vi "Run 2 Averaged History.vi"(11 "2D Run Data":dbl[][](array[numeric])=[[1.0, 11.0], [2.0, 12.0], [3.0, 13.0], [4.0, 14.0], [5.0, 15.0], [6.0, 16.0], [7.0, 17.0], [8.0, 18.0], [9.0, 19.0], [10.0, 20.0], [2.0, 12.0], [3.0, 13.0], [4.0, 14.0], [5.0, 15.0], [6.0, 16.0], [7.0, 17.0], [8.0, 18.0], [9.0, 19.0], [10.0, 20.0], [11.0, 21.0]]) -> (3 "Data 2D IN out":dbl[](array[numeric]))   [LabVIEW 2011]
panel:
  out "Averaged Integration Spectra":dbl[][](array[numeric])=[[1.5, 11.5], [2.5, 12.5], [3.5, 13.5], [4.5, 14.5], [5.5, 15.5], [6.5, 16.5], [7.5, 17.5], [8.5, 18.5], [9.5, 19.5], [10.5, 20.5]]
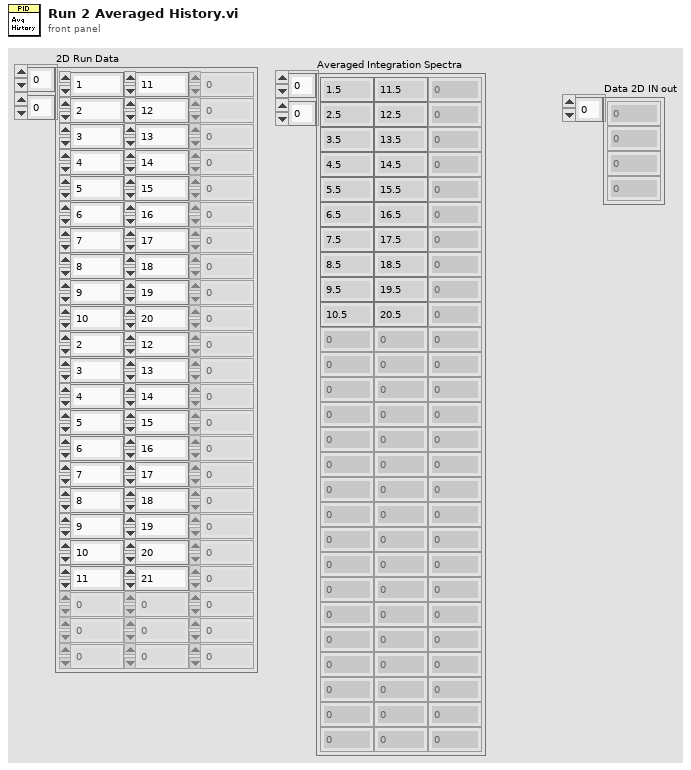
[diagram p1: front panel]
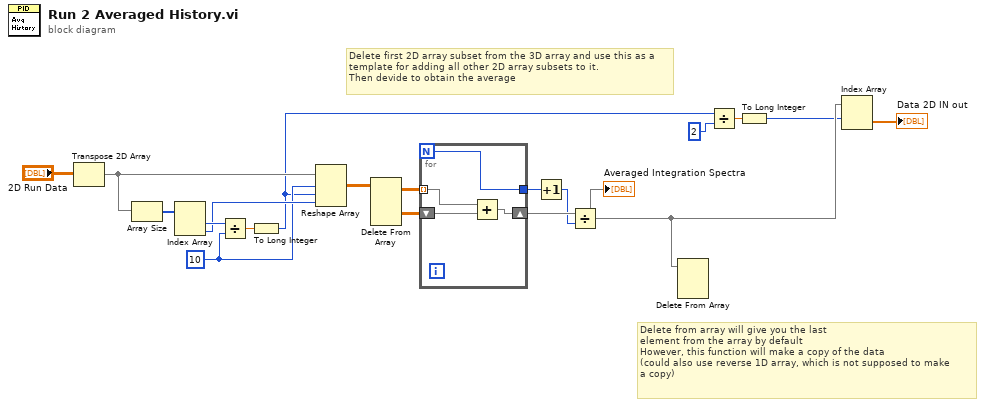
[diagram p0: block diagram]
diagram:
  w7 = 10 ("y")
  # "Delete from array will give you the last \nelement from the array by default\nHowever, this function will make a copy of the data\n(could also use reverse 1D array, which is not supposed to make\na copy)"
  # "Delete first 2D array subset from the 3D array and use this as a\ntemplate for adding all other 2D array subsets to it.\nThen devide to obtain the average"
  n1 = Transpose 2D Array(2D array="2D Run Data") -> (transposed array=w8:dbl[][])
  n2 = Array Size(array=w8) -> (size(s)=w19:i32[])
  n3 = Index Array(array=w19) -> (element #1=w18:i32, element #2=w16:i32)  [unwired: 2 in]
  n4 = Divide(x=w18, y=w7) -> (x/y=w17:dbl)
  n5 = To Long Integer(number=w17) -> (32bit integer=w5:i32)
  n6 = Reshape Array(w8, w7, w5, w16) -> (w12:dbl[][][])
  n7 = Delete From Array(array=w12) -> (deleted portion=w11:dbl[][], array with subset deleted=w10:dbl[][][])  [unwired: 4 in]
  n8 = for {
    N -> [w20]
    tunnel: w10 -> [w23] mode=indexing
    shift-right: [w21] -> w14
    shift-left: w11 -> [w22]
    tunnel: [w20] -> w15
    n9 = Add(x=w23, y=w22) -> (x+y=w21:dbl[][])
  }
  n10 = Increment(x=w15) -> (x+1=w13:i32)
  n11 = Divide(x=w14, y=w13) -> (x/y=w6:dbl[][])
  "Averaged Integration Spectra" <- w6
  n12 = Delete From Array(array=w6) -> ()  [unwired: 3 in, 2 out]
  n13 = Divide(x=w5, y=2) -> (x/y=w3:dbl)
  n14 = To Long Integer(number=w3) -> (32bit integer=w2:i32)
  n15 = Index Array(array=w6, index (row)=w2) -> (element=→"Data 2D IN out":dbl[])  [unwired: 1 in]
